vi "Get General Configuration.vi"(8 "error in (no error)":errorcluster, 11 "Ethernet in":refnum<class "ENET_BS1201.lvclass">) -> (0 "error out":errorcluster, 1 "Configuration Error?":bool, 2 "Protocol (Legacy)":T1=enum."Ethernet", 3 "Ethernet out":refnum<class "ENET_BS1201.lvclass">, 4 "Cell Inhibit Enable":bool)   [LabVIEW 2021, in "BS120x Driver.lvlib" / "ENET_BS1201.lvclass"]
doc: "Retrieve Battery Simulator 1200 general settings.\n(c) 2019 Bloomy Controls, Inc. All rights reserved."
uses:
  ENET_BS1201.lvclass
  TypeDefs/Protocol.ctl
  ENET_BS1201.lvclass/ENET_BS1201.ctl
  BS120x.lvclass
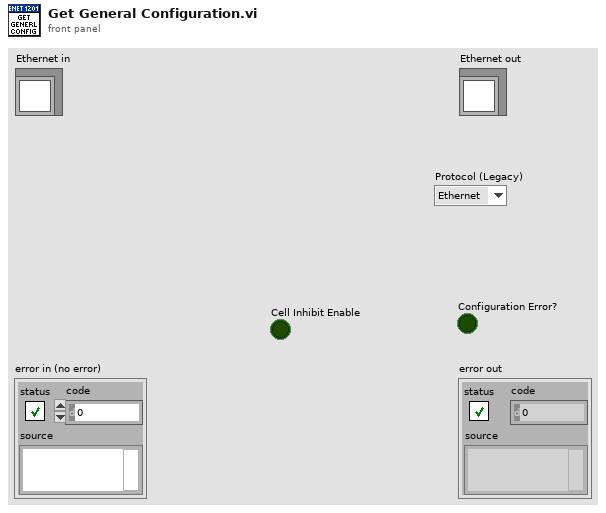
[diagram p1: front panel]
types:
  T1 = typedef "BS120x Driver.lvlib/BS120x.lvclass/Protocol.ctl" = enum16{"CAN", "Ethernet"}
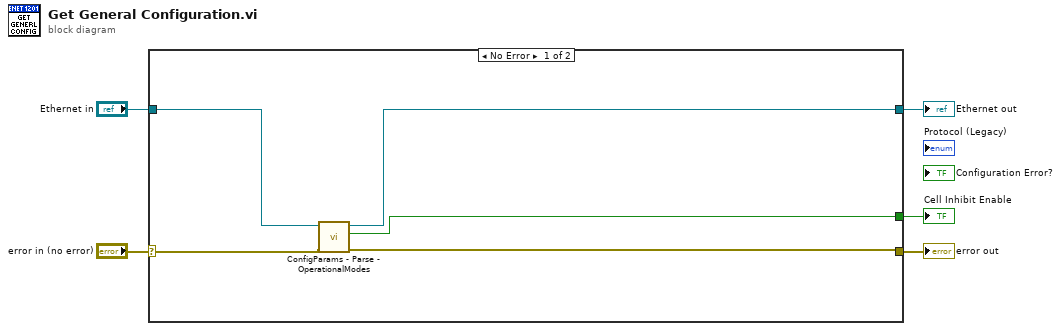
[diagram p0: block diagram]
diagram:
  n1 = case shown="No Error" "error in (no error)" {
    selector: "error in (no error)" -> [w10 w12]
    tunnel: [w9 w12] -> w4
    tunnel: [w7 w11] -> w2
    tunnel: "Ethernet in" -> [w8 w11]
    tunnel: [w6 _] -> w1
    frame No Error {
      n2 = call-dynamic "ConfigParams - Parse - OperationalModes.vi"("error in (no error)"=w10, "Ethernet in"=w8) -> ("error out"=w9:errorcluster, "CellInhibitEnable"=w6:bool, "Ethernet out"=w7:refnum<class "ENET_BS1201.lvclass">)  [unwired: 7 in]
    }
    frame Error {
    }
  }
  "error out" <- w4
  "Ethernet out" <- w2
  "Cell Inhibit Enable" <- w1
